vi "Register Configuration and Results.vi"(8 "error in (no error)":errorcluster, 11 "gRPC ID":T1) -> (0 "error out":errorcluster, 3 "gRPC ID Out":T1)   [LabVIEW 2020, in "LineRegulation.lvlib"]
uses:
  LineRegulation.lvlib
  <vilib>/gRPC/LabVIEW gRPC Library/Shared/grpcId.ctl
  Measurement Configuration.ctl
  Measurement Results.ctl
  <vilib>/gRPC/LabVIEW gRPC Library/grpc-lvsupport-release.lvlib
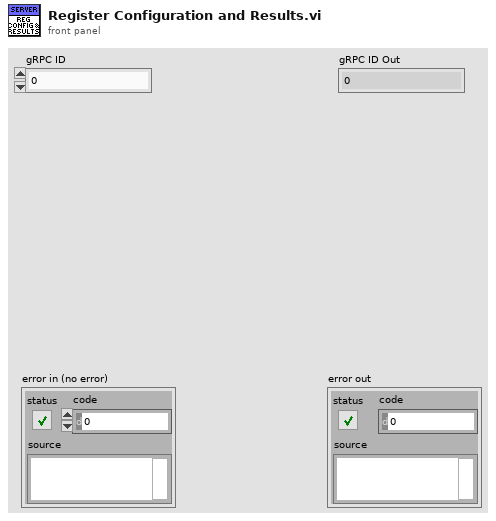
[diagram p1: front panel]
types:
  T1 = typedef "grpc-lvsupport-release.lvlib/grpcId.ctl" = u64
  T2 = typedef "LineRegulation.lvlib/Measurement Results.ctl" = cluster{"Array out":dbl[]}
  T3 = typedef "LineRegulation.lvlib/Measurement Configuration.ctl" = cluster{"Array in":dbl[]}
  T4 = typedef "grpc-lvsupport-release.lvlib/Message Metadata.ctl" = cluster{"Version":i32, "Name":string, "Type Url":string, "Elements":T5[]}
  T5 = typedef "grpc-lvsupport-release.lvlib/Message Element Metadata.ctl" = cluster{"Embedded Message Name":string, "Protobuf Index":i32, "MessageElementType":T6, "Repeated":bool}
  T6 = typedef "grpc-lvsupport-release.lvlib/Message Element Type.ctl" = enum32{"Int32Value", "FloatValue", "DoubleValue", "BoolValue", "StringValue", "MessageValue", "Int64Value", "UInt32Value", "UInt64Value", "EnumValue", "Bytes", "Fixed64", "Fixed32", "SFixed64", "SFixed32", "SInt64", "SInt32"}
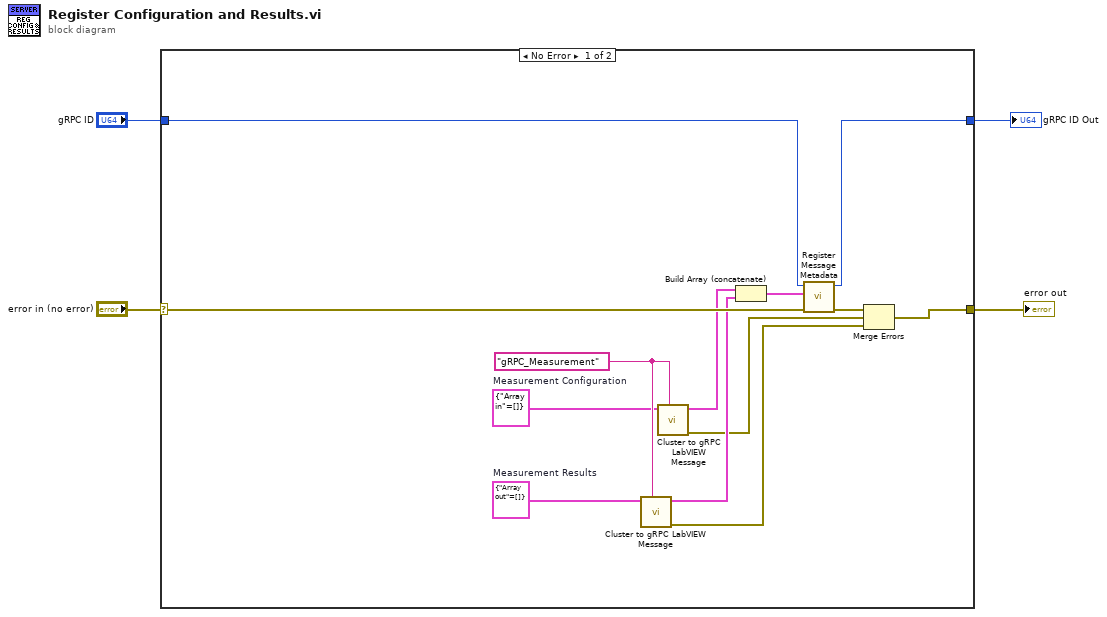
[diagram p0: block diagram]
diagram:
  n1 = case shown="No Error" "error in (no error)" {
    selector: "error in (no error)" -> [w16 w19]
    tunnel: [w9 w18] -> w1
    tunnel: [w12 w19] -> w4
    tunnel: "gRPC ID" -> [w8 w18]
    frame No Error {
      w5 = T2 {"Array out"=[]}  # Measurement Results
      w6 = T3 {"Array in"=[]}  # Measurement Configuration
      w7 = "gRPC_Measurement" ("Package Name")
      n2 = call <vilib>:"Cluster to gRPC LabVIEW Message.vi"("Package Name"=w7, "Cluster"=w5) -> ("error out"=w11:errorcluster, "gRPC Message Metadata []"=w14:T4[])  [unwired: 8 in]
      n3 = call <vilib>:"Cluster to gRPC LabVIEW Message.vi"("Package Name"=w7, "Cluster"=w6) -> ("error out"=w10:errorcluster, "gRPC Message Metadata []"=w15:T4[])  [unwired: 8 in]
      n4 = Build Array (concatenate)(w15, w14) -> (w13:T4[])
      n5 = call <vilib>:"Register Message Metadata.vi"("error in"=w16, "Messages"=w13, "gRPCid in"=w8) -> ("error out"=w17:errorcluster, "gRPCid out"=w9:T1)  [unwired: 7 in]
      n6 = Merge Errors(w17, w10, w11) -> (w12:errorcluster)
    }
    frame Error {
    }
  }
  "error out" <- w4
  "gRPC ID Out" <- w1
